vi "Retrieve.vi"(8 "error in (no error)":errorcluster, 11 "MatchData in":refnum<class "MatchData.lvclass">) -> (0 "error out":errorcluster, 1 "Quem joga":string, 2 "Tabuleiro":T1, 3 "MatchData out":refnum<class "MatchData.lvclass">)   [LabVIEW 2018, in "MatchData.lvclass"]
uses:
  MatchData.lvclass
  controls/Tabuleiro.ctl
  MatchData.lvclass/MatchData.ctl
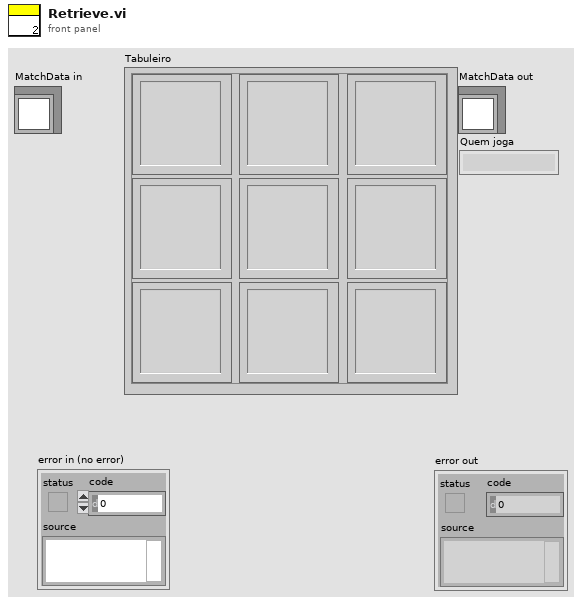
[diagram p1: front panel]
types:
  T1 = typedef "Tabuleiro.ctl" = cluster{"(0,0)":string, "(1,0)":string, "(0,1)":string, "(1,1)":string, "(2,0)":string, "(1,2)":string, "(2,2)":string, "(0,2)":string, "(2,1) ":string}
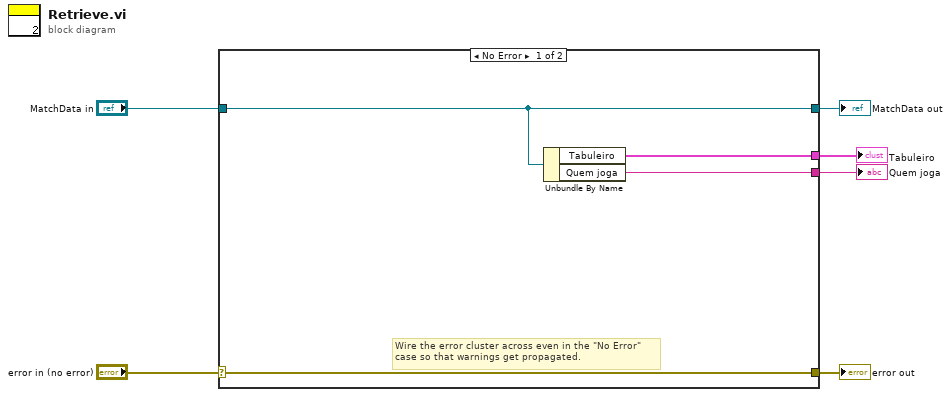
[diagram p0: block diagram]
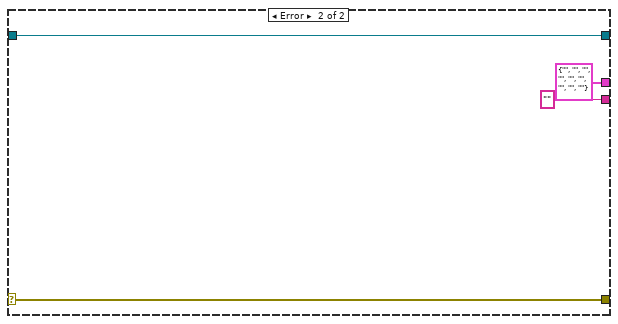
[diagram p2: hidden frame]
diagram:
  n1 = case shown="No Error" "error in (no error)" {
    selector: "error in (no error)" -> [w10 w14]
    tunnel: [w10 w14] -> w5
    tunnel: [w9 w13] -> w3
    tunnel: "MatchData in" -> [w9 w13]
    tunnel: [w8 "" ("Quem joga")] -> w2
    tunnel: [w7 T1 {"(0,0)"="", "(1,0)"="", "(0,1)"="", "(1,1)"="", "(2,0)"="", "(1,2)"="", "(2,2)"="", "(0,2)"="", "(2,1) "=""} ("Tabuleiro")] -> w1
    frame No Error {
      # "Wire the error cluster across even in the \"No Error\"\ncase so that warnings get propagated."
      n2 = Unbundle By Name(w9) -> ("Tabuleiro"=w7:T1, "Quem joga"=w8:string)
    }
    frame Error {
    }
  }
  "error out" <- w5
  "MatchData out" <- w3
  "Tabuleiro" <- w1
  "Quem joga" <- w2
